vi "Initialize  (iSUB) (SubVI).vi"(6 "Image Size":T1={"Height"=2048, "Width"=2048}, 11 "REF IN":T2) -> (0 "Exp. Status":string="Camera Connected", 1 "OK?":bool, 3 "REF OUT":T2)   [LabVIEW 2015]
uses:
  Controls (HOST)/Data to Disk Bundle.ctl
  Controls (HOST)/Image Queue Bundle.ctl
  Controls (HOST)/REF.ctl
  Controls (HOST)/Image Size.ctl
  Controls (HOST)/FPGA REF (MWT).ctl
  Controls (HOST)/FPGA REF (iSUB).ctl
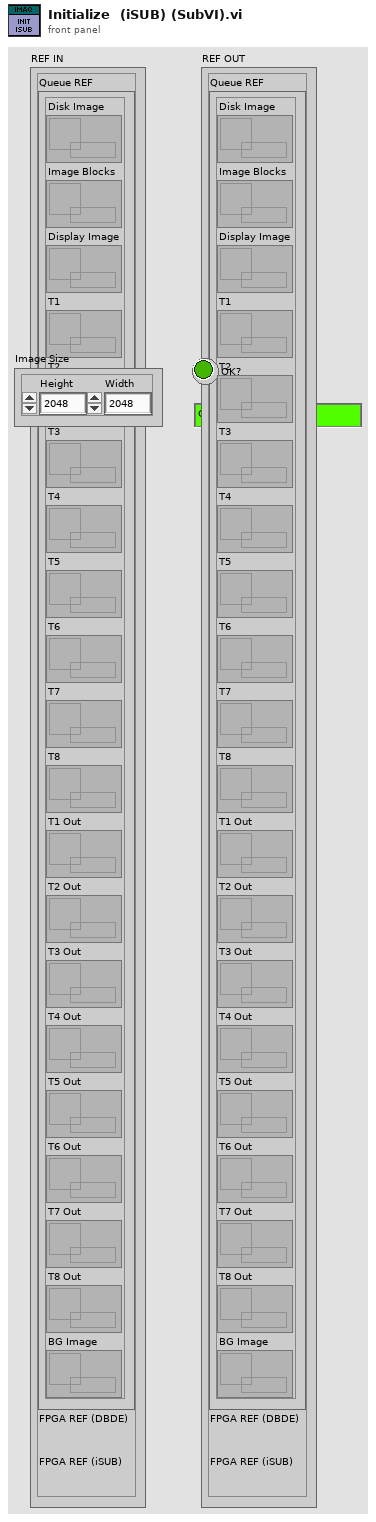
[diagram p1: front panel]
types:
  T1 = typedef "Image Size.ctl" = cluster{"Height":u16, "Width":u16}
  T2 = typedef "REF.ctl" = cluster{"Queue REF":T3, "FPGA REF (DBDE)":T4, "FPGA REF (iSUB)":T5}
  T3 = typedef "Image Queue Bundle.ctl" = cluster{"Disk Image":refnum<queue>, "Image Blocks":refnum<queue>, "Display Image":refnum<queue>, "T1":refnum<queue>, "T2":refnum<queue>, "T3":refnum<queue>, "T4":refnum<queue>, "T5":refnum<queue>, "T6":refnum<queue>, "T7":refnum<queue>, "T8":refnum<queue>, "T1 Out":refnum<queue>, "T2 Out":refnum<queue>, "T3 Out":refnum<queue>, "T4 Out":refnum<queue>, "T5 Out":refnum<queue>, "T6 Out":refnum<queue>, "T7 Out":refnum<queue>, "T8 Out":refnum<queue>, "BG Image":refnum<queue>}
  T4 = typedef "FPGA REF (MWT).ctl" = refnum<k20>
  T5 = typedef "FPGA REF (iSUB).ctl" = refnum<k20>
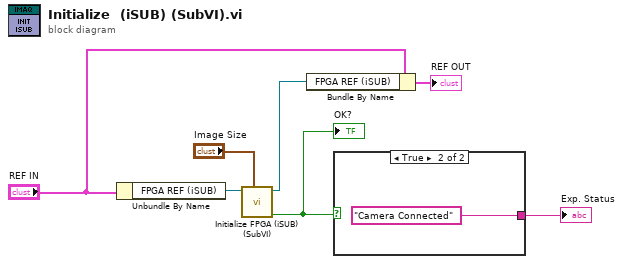
[diagram p0: block diagram]
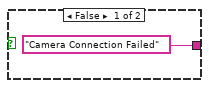
[diagram p2: hidden frame]
diagram:
  n1 = Unbundle By Name("REF IN") -> ("FPGA REF (iSUB)"=w7:T5)
  n2 = call "Initialize FPGA (iSUB) (SubVI).vi"("Image Size"="Image Size", "FPGA REF (iSUB) IN"=w7) -> ("Camera OK?"=w5:bool, "FPGA REF (iSUB) OUT"=w2:T5)  [unwired: 8 in]
  "OK?" <- w5
  n3 = Bundle By Name(cluster="REF IN", "FPGA REF (iSUB)"=w2) -> (→"REF OUT":T2)
  n4 = case shown="True" w5 {
    tunnel: ["Camera Connection Failed" "Camera Connected"] -> w6
    frame False {
    }
    frame True {
    }
  }
  "Exp. Status" <- w6
